vi "Get Int.vi"(8 "error in (no error)":errorcluster, 11 "IInt in":refnum<class "IInt.lvclass">) -> (0 "error out":errorcluster, 2 "Int":i32, 3 "IInt out":refnum<class "IInt.lvclass">)   [LabVIEW 2009, in "IInt.lvclass"]
uses:
  IInt.lvclass
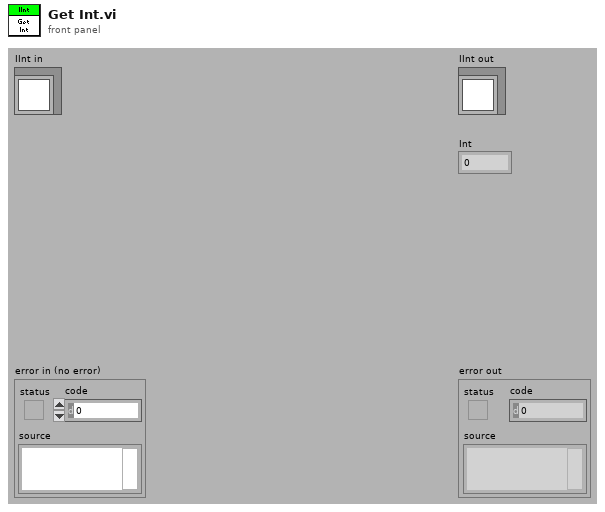
[diagram p1: front panel]
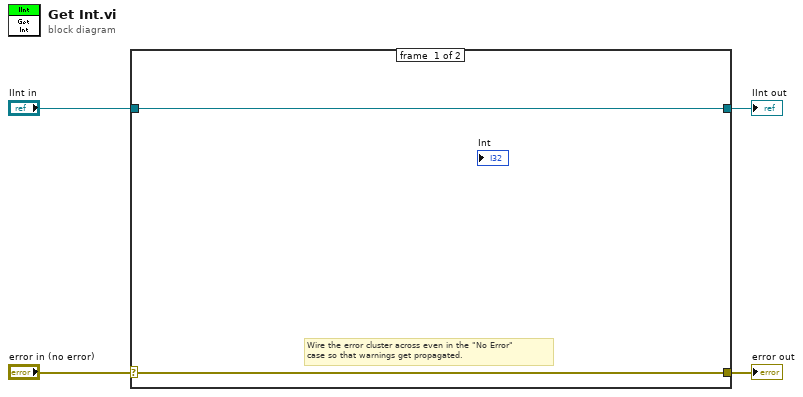
[diagram p0: block diagram]
diagram:
  n1 = case shown="No Error" "error in (no error)" {
    selector: "error in (no error)" -> [w5 w8]
    tunnel: [w5 w8] -> w3
    tunnel: [w6 w7] -> w1
    tunnel: "IInt in" -> [w6 w7]
    frame #0 {
      # "Wire the error cluster across even in the \"No Error\"\ncase so that warnings get propagated."
    }
    frame #1 {
    }
  }
  "error out" <- w3
  "IInt out" <- w1
